vi "存档数据添加时间和结果.vi"(10 "结果":bool, 11 "待写入数据":string[](array[string])) -> (3 "添加了时间，结果的存档数据":string[](array[string]))   [LabVIEW 2014]
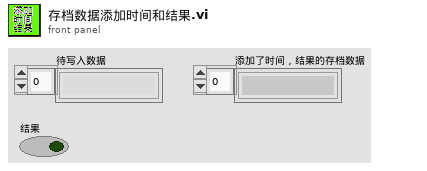
[diagram p1: front panel]
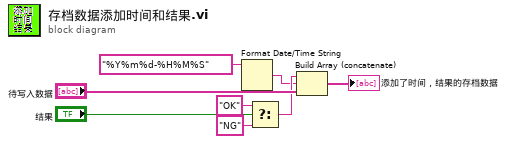
[diagram p0: block diagram]
diagram:
  n1 = Format Date/Time String(time format string (%c)="%Y%m%d-%H%M%S") -> (date/time string=w1:string)  [unwired: 2 in]
  n2 = Select(t="OK", s="结果", f="NG") -> (s? t:f=w2:string)
  n3 = Build Array (concatenate)(w2, w1, "待写入数据") -> (→"添加了时间，结果的存档数据":string[])
